vi "mbtester_main.vi"() -> ()   [LabVIEW 2012]
uses:
  source/TSKMGR_TaskManager/mbTest_main_gui_states.ctl
  <vilib>/Utility/miscctls.llb/LVRectTypeDef.ctl
  <vilib>/Utility/miscctls.llb/LVRowAndColumnTypeDef.ctl
  <vilib>/Utility/miscctls.llb/LVRowAndColumnUnsignedTypeDef.ctl
  source/APP_AppControl/APP_AppControl.lvlib
  source/TSKMGR_TaskManager/TSKMGR_TaskManager.lvlib
  source/FP_FrontPanel/FP_FrontPanel.lvlib
  source/MBUS_Modbus/MBUS_Modbus.lvlib
  source/MBT_ModbusTester/MBT_ModbusTester.lvlib
panel:
  in  "Data Format":u16(ring) items=["Decimal", "Hexadecimal", "String"]
  in  "Multicolumn Listbox":i32(listbox)
  in  "btnClear":bool
  in  "btnSaveToFile":bool
  in  "btnDisconnect":bool
  out "isConnected":bool
  in  "btnConnect":bool
  in  "Number of Regs.":u16 max=125
  in  "Starting Reg.":u16
  in  "Port":u16
  in  "IP Address":string
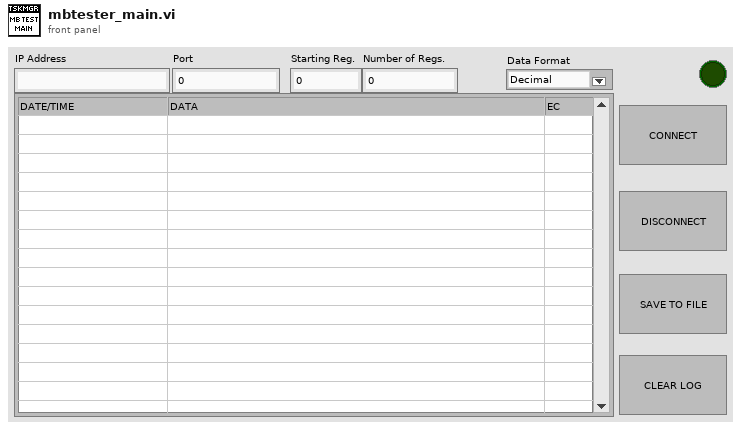
[diagram p1: front panel]
types:
  T1 = typedef "TSKMGR_TaskManager.lvlib/mbTest_main_gui_states.ctl" = enum16{"INIT", "IDLE", "CONNECT", "OPERATE", "DISCONNECT", "CLEAR", "EXIT_APP", "SAVE"}
  T2 = enum8{"Enabled", "Disabled", "Disabled and Grayed Out"}
  T3 = cluster{"isConnected":bool, "connection ID":refnum<k5>, "IP Address":string, "Port":dbl}
  T4 = typedef "LVRectTypeDef.ctl" = cluster{"Left":i16, "Top":i16, "Right":i16, "Bottom":i16}
  T5 = typedef "LVRowAndColumnUnsignedTypeDef.ctl" = cluster{"Row":u32, "Column":u32}
  T6 = typedef "LVRowAndColumnTypeDef.ctl" = cluster{"Row":i32, "Column":i32}
  T7 = cluster{"App_EvtCmds":enum16{"CLOSE_APP"}, "variant":variant}
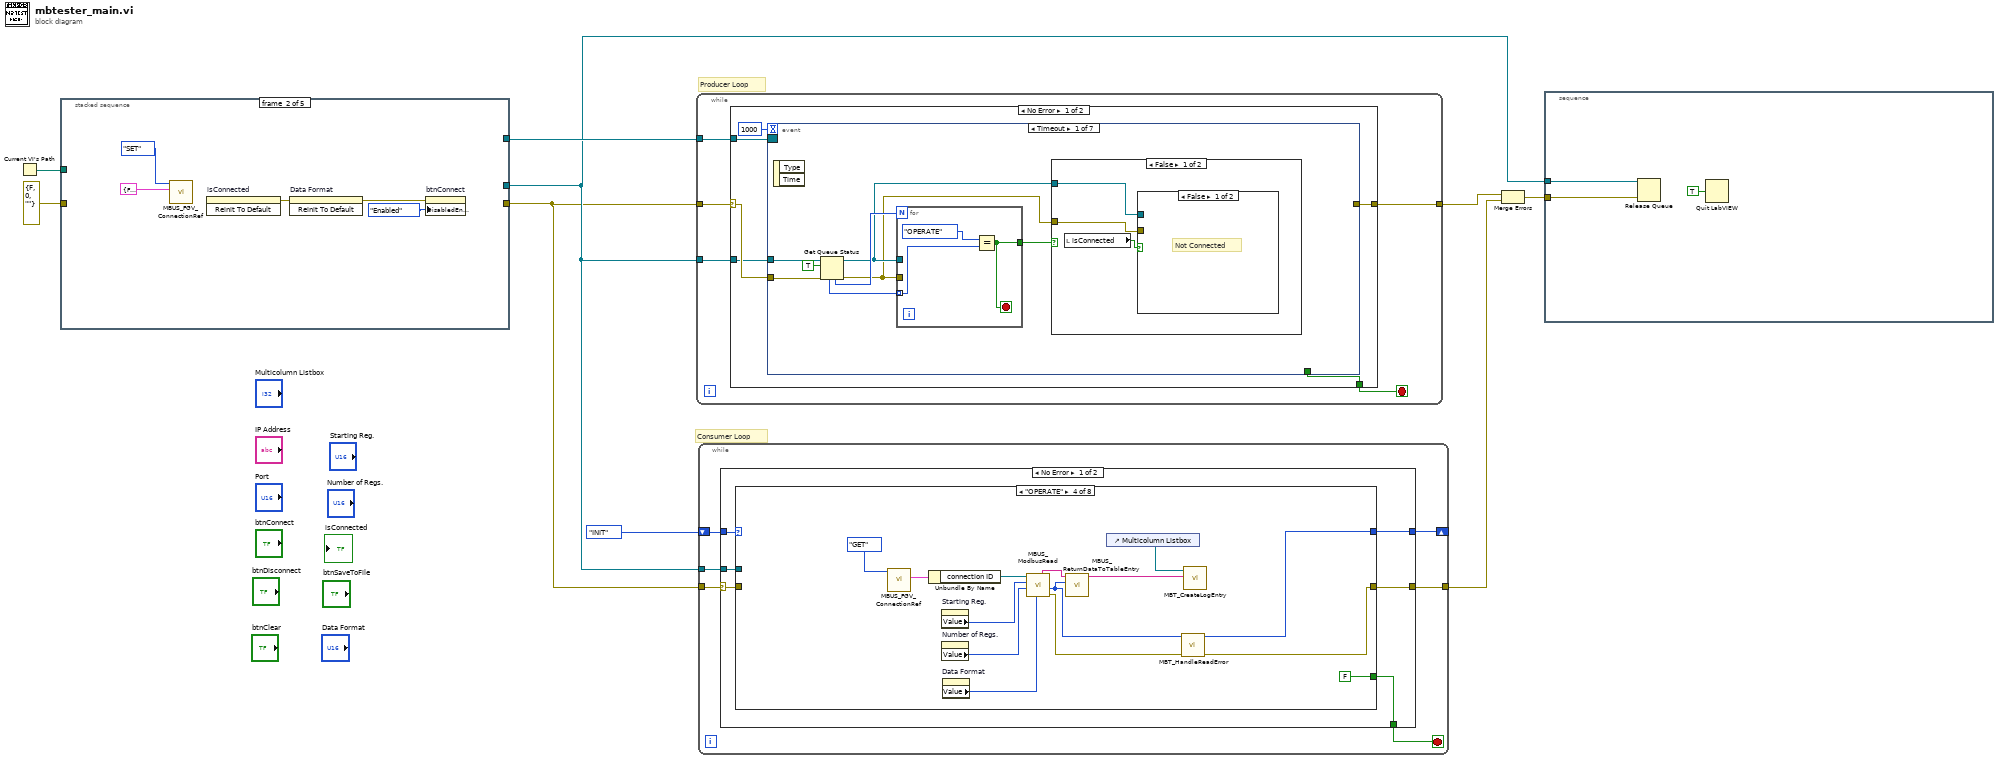
[diagram p0: block diagram]
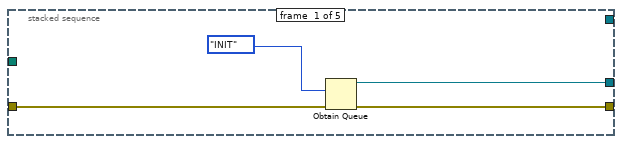
[diagram p2: hidden frame]
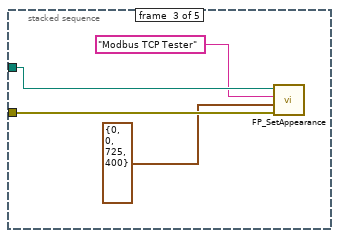
[diagram p3: hidden frame]
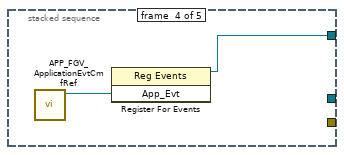
[diagram p4: hidden frame]
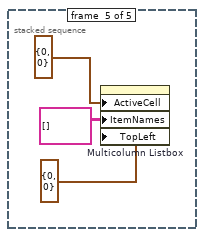
[diagram p5: hidden frame]
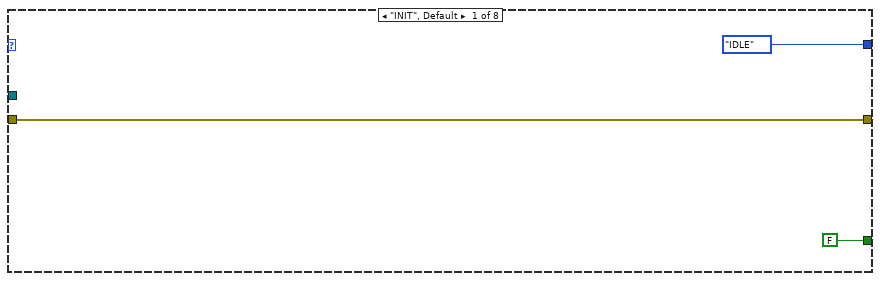
[diagram p6: hidden frame]
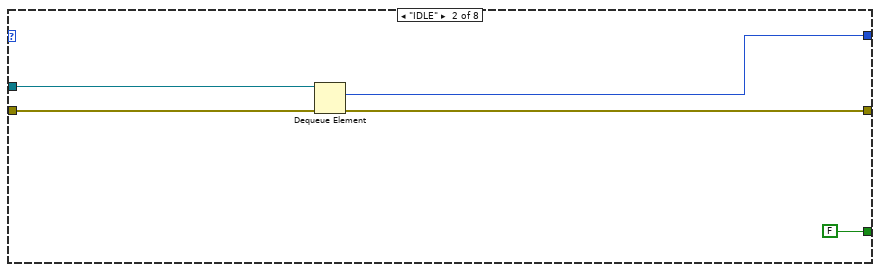
[diagram p7: hidden frame]
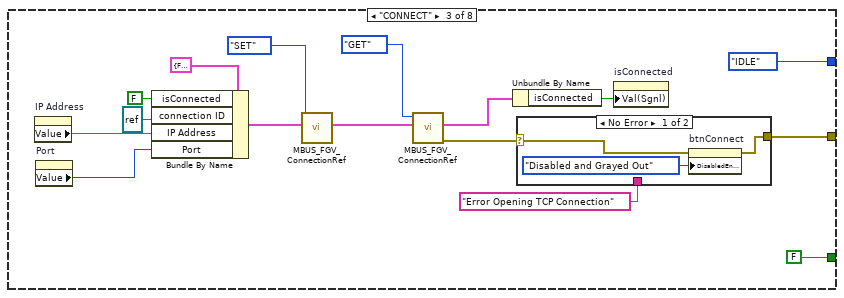
[diagram p8: hidden frame]
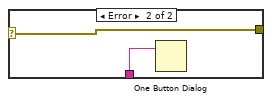
[diagram p9: hidden frame]
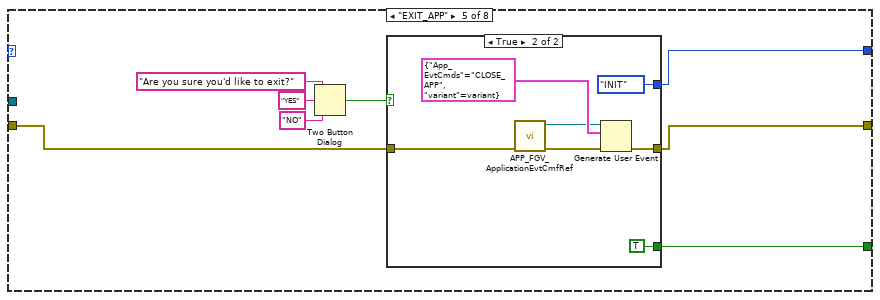
[diagram p10: hidden frame]
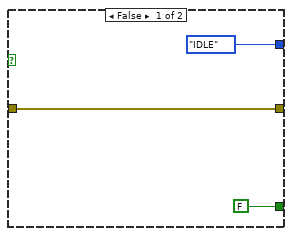
[diagram p11: hidden frame]
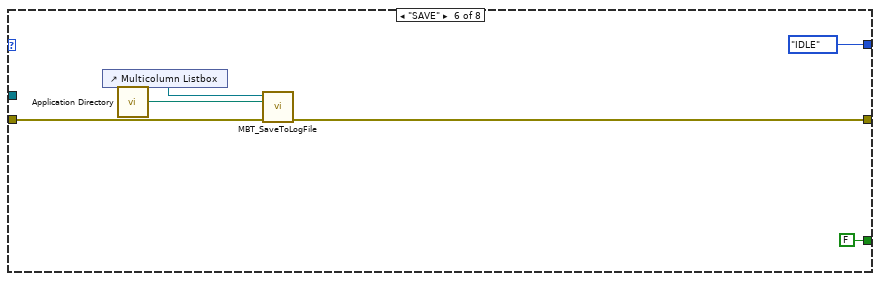
[diagram p12: hidden frame]
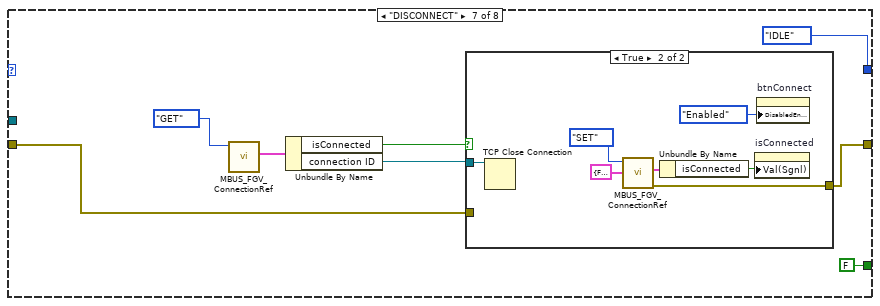
[diagram p13: hidden frame]
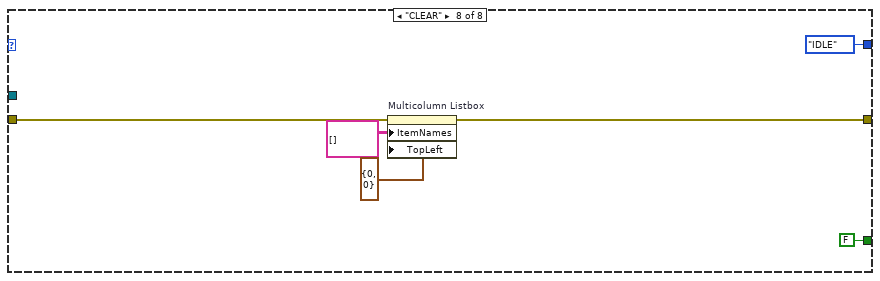
[diagram p15: hidden frame]
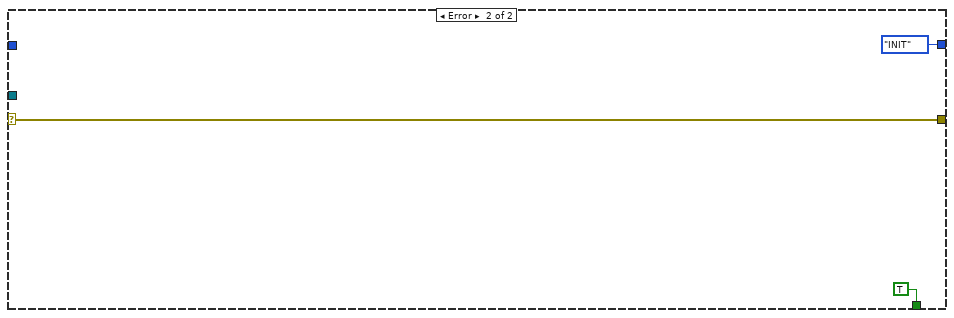
[diagram p16: hidden frame]
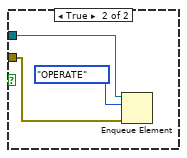
[diagram p17: hidden frame]
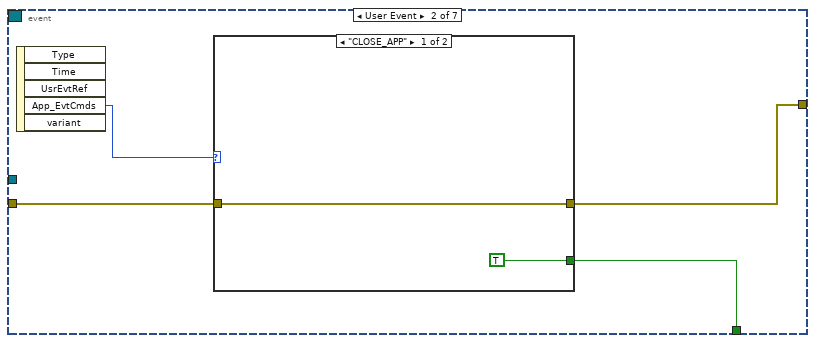
[diagram p19: hidden frame]
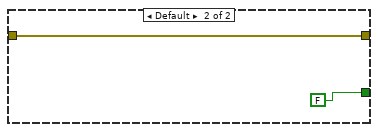
[diagram p20: hidden frame]
diagram:
  # "Consumer Loop"
  # "Producer Loop"
  n1 = Current VI's Path() -> (path=w2:path)
  n2 = stacked-sequence {
    tunnel: [_ _ _ w23 _] -> w9
    tunnel: [w10 _ _ _ _] -> w1
    tunnel: [w11 _ _ _ _] -> w3
    tunnel: errorcluster {"status"=FALSE, "code"=0, "source"=""} ("error in (no error)") -> [w13 _ w22 _ _]
    tunnel: w2 -> [_ _ w21 _ _]
    frame #0 {
      n3 = Obtain Queue(element data type=mbTest_main_gui_states."INIT", error in (no error)=w13) -> (queue out=w11:refnum<queue>, error out=w10:errorcluster)  [unwired: 3 in, 1 out]
    }
    frame #1 {
      n4 = call "MBUS_FGV_ConnectionRef.vi"("ConnectionRefIn"=T3 {"isConnected"=FALSE, "connection ID"=refnum, "IP Address"="", "Port"=0.0}, "CMD"=enum16{"GET", "SET"}."SET") -> ()  [unwired: 8 in, 2 out]
      n5 = invoke on="isConnected" class="Bool" method="Reinit To Default"() -> (error out=w14:errorcluster)  [unwired: 3 in, 2 out]
      n6 = invoke on="Data Format" class="Ring (strict)" method="Reinit To Default"(error in=w14) -> (error out=w15:errorcluster)  [unwired: 2 in, 2 out]
      n7 = property on="btnConnect" class="Bool"(error in=w15, "DisabledEnum"=T2."Enabled" ("Disabled")) -> ()  [unwired: 1 in, 2 out]
    }
    frame #2 {
      n8 = call "FP_SetAppearance.vi"("error in (no error)"=w22, "Front Panel Window:Window Bounds 2"=T4 {"Left"=0, "Top"=0, "Right"=725, "Bottom"=400}, "Front Panel Window:Title"="Modbus TCP Tester", "vi path"=w21) -> ()  [unwired: 7 in, 1 out]
    }
    frame #3 {
      n9 = call "APP_FGV_ApplicationEvtCmfRef.vi"() -> ("App_Evt"=w24:refnum<user-event>)  [unwired: 10 in, 1 out]
      n10 = register-events(w24) -> (reference out=w23:refnum<event-registration>)  [unwired: 2 in, 1 out]
    }
    frame #4 {
      n11 = property on="Multicolumn Listbox" class="MCListbox (strict)"("ActiveCell"=T6 {"Row"=0, "Column"=0} ("Active Cell:Active Cell"), "ItemNames"=string[][] [] ("Item Names"), "TopLeft"=T5 {"Row"=0, "Column"=0} ("Top Left Visible Cell")) -> ()  [unwired: 2 in, 2 out]
    }
  }
  n12 = while {
    tunnel: w9 -> [w32]
    tunnel: w1 -> [w31]
    tunnel: [w29] -> w4
    tunnel: w3 -> [w28]
    stop <- w30 stop-if-true
    n13 = case shown="No Error" w31 {
      selector: w31 -> [w37 w86]
      tunnel: w32 -> [w38 _]
      tunnel: [w34 TRUE] -> w30
      tunnel: [w36 w86] -> w29
      tunnel: w28 -> [w35 _]
      frame No Error {
        n14 = event shown="[0] Timeout" {
          selector: w38 -> [_ _ _ _ _ _ _]
          dyn-events: _ -> [_ _ _ _ _ _ _]
          timeout: 1000 -> [_ _ _ _ _ _ _]
          tunnel: w37 -> [w45 w57 w65 w70 w77 w79 w83]
          tunnel: [_ w56 _ _ w74 _ _] -> w36
          tunnel: w35 -> [w46 _ w66 w72 w76 w80 w84]
          tunnel: [_ w58 _ FALSE _ _ _] -> w34
          event Timeout {
            n15 = event-data() -> ()  [unwired: 1 in, 2 out]
            n16 = Get Queue Status(queue=w46, return elements? (F)=TRUE, error in (no error)=w45) -> (queue out=w40:refnum<queue>, error out=w39:errorcluster, # elements in queue=w44:i32, elements=w43:T1[])  [unwired: 4 out]
            n17 = for {
              N: w44 -> [_]
              tunnel: w43 -> [w49] mode=indexing
              tunnel: [w47] -> w41
              tunnel: w40 -> [_]
              tunnel: w39 -> [_]
              stop <- w47 stop-if-true
              n18 = Equal?(x=mbTest_main_gui_states."OPERATE", y=w49) -> (x = y?=w47:bool)
            }
            n19 = case shown="False" w41 {
              tunnel: w40 -> [w51 _]
              tunnel: w39 -> [w50 _]
              frame False {
                n20 = local read "isConnected"() -> (w52:bool)
                n21 = case shown="False" w52 {
                  tunnel: w51 -> [_ w54]
                  tunnel: w50 -> [_ w53]
                  frame False {
                    # "Not Connected"
                  }
                  frame True {
                    n22 = Enqueue Element(queue=w54, element=mbTest_main_gui_states."OPERATE", error in (no error)=w53) -> ()  [unwired: 1 in, 3 out]
                  }
                }
              }
              frame True {
                # "Operate already in queue"
              }
            }
          }
          event User Event {
            n23 = event-data() -> ("App_EvtCmds"=w59:enum16{"CLOSE_APP"})  [unwired: 1 in, 4 out]
            n24 = case shown="\"CLOSE_APP\"" w59 {
              tunnel: [TRUE FALSE] -> w58
              tunnel: [w60 w62] -> w56
              tunnel: w57 -> [w60 w62]
              frame "CLOSE_APP" {
              }
              frame Default {
              }
            }
          }
          event "btnClear": Value Change {
            n25 = event-data() -> ("CtlRef"=w67:refnum<vi>)  [unwired: 1 in, 4 out]
            n26 = Enqueue Element(queue=w66, element=mbTest_main_gui_states."CLEAR", error in (no error)=w65) -> ()  [unwired: 1 in, 3 out]
            n27 = invoke class="Bool" method="Reinit To Default"(reference=w67) -> ()  [unwired: 2 in, 3 out]
          }
          event "btnConnect": Value Change {
            n28 = event-data() -> ("CtlRef"=w69:refnum<vi>)  [unwired: 1 in, 4 out]
            n29 = Enqueue Element(queue=w72, element=mbTest_main_gui_states."CONNECT", error in (no error)=w70) -> ()  [unwired: 1 in, 3 out]
            n30 = invoke class="Bool" method="Reinit To Default"(reference=w69) -> ()  [unwired: 2 in, 3 out]
          }
          event Panel Close? {
            n31 = event-data() -> ()  [unwired: 1 in, 3 out]
            n32 = Enqueue Element At Opposite End(queue=w76, element=mbTest_main_gui_states."EXIT_APP", error in (no error)=w77) -> (error out=w74:errorcluster)  [unwired: 1 in, 2 out]
            n33 = event-data("Discard?"=TRUE) -> ()  [unwired: 1 in, 1 out]
          }
          event "btnDisconnect": Value Change {
            n34 = event-data() -> ("CtlRef"=w78:refnum<vi>)  [unwired: 1 in, 4 out]
            n35 = Enqueue Element(queue=w80, element=mbTest_main_gui_states."DISCONNECT", error in (no error)=w79) -> ()  [unwired: 1 in, 3 out]
            n36 = invoke class="Bool" method="Reinit To Default"(reference=w78) -> ()  [unwired: 2 in, 3 out]
          }
          event "btnSaveToFile": Value Change {
            n37 = event-data() -> ("CtlRef"=w85:refnum<vi>)  [unwired: 1 in, 4 out]
            n38 = Enqueue Element(queue=w84, element=mbTest_main_gui_states."SAVE", error in (no error)=w83) -> ()  [unwired: 1 in, 3 out]
            n39 = invoke class="Bool" method="Reinit To Default"(reference=w85) -> ()  [unwired: 2 in, 3 out]
          }
        }
      }
      frame Error {
      }
    }
  }
  n40 = while {
    tunnel: w1 -> [w93]
    tunnel: w3 -> [w91]
    shift-right: [w89] -> _
    shift-left: mbTest_main_gui_states."INIT" -> [w90]
    tunnel: [w88] -> w5
    stop <- w92 stop-if-true
    n41 = case shown="No Error" w93 {
      selector: w93 -> [w97 w190]
      tunnel: [w95 TRUE] -> w92
      tunnel: w91 -> [w94 _]
      tunnel: w90 -> [w99 _]
      tunnel: [w98 mbTest_main_gui_states."INIT"] -> w89
      tunnel: [w96 w190] -> w88
      frame No Error {
        n42 = case shown="\"OPERATE\"" w99 {
          tunnel: [mbTest_main_gui_states."IDLE" w104 mbTest_main_gui_states."IDLE" ("f") w129 w144 mbTest_main_gui_states."IDLE" mbTest_main_gui_states."IDLE" mbTest_main_gui_states."IDLE"] -> w98
          tunnel: w97 -> [w101 w106 _ _ w146 w164 w167 w186]
          tunnel: [w101 w103 w110 w130 w145 w163 w169 w185] -> w96
          tunnel: [FALSE FALSE FALSE FALSE w143 FALSE FALSE FALSE] -> w95
          tunnel: w94 -> [_ w105 _ _ _ _ _ _]
          frame "INIT", Default {
          }
          frame "IDLE" {
            n43 = Dequeue Element(queue=w105, error in (no error)=w106) -> (element=w104:T1, error out=w103:errorcluster)  [unwired: 1 in, 2 out]
          }
          frame "CONNECT" {
            n44 = property on="IP Address" class="Str"() -> ("Value"=w116:string)  [unwired: 2 in, 2 out]
            n45 = property on="Port" class="DigNum (strict)"() -> ("Value"=w115:u16)  [unwired: 2 in, 2 out]
            n46 = Bundle By Name(cluster=T3 {"isConnected"=FALSE, "connection ID"=refnum, "IP Address"="", "Port"=0.0} ("ConnectionRefIn"), "isConnected"=FALSE, "connection ID"=refnum<k5> refnum, "IP Address"=w116, "Port"=w115) -> (w119:T3)
            n47 = call "MBUS_FGV_ConnectionRef.vi"("ConnectionRefIn"=w119, "CMD"=enum16{"GET", "SET"}."SET") -> ("ConnectionRefOut"=w118:T3)  [unwired: 8 in, 1 out]
            n48 = call "MBUS_FGV_ConnectionRef.vi"("ConnectionRefIn"=w118, "CMD"=enum16{"GET", "SET"}."GET") -> ("error out"=w111:errorcluster, "ConnectionRefOut"=w117:T3)  [unwired: 8 in]
            n49 = Unbundle By Name(w117) -> ("isConnected"=w108:bool)
            n50 = case shown="No Error" w111 {
              selector: w111 -> [w125 w127]
              tunnel: [w126 w127] -> w110
              tunnel: "Error Opening TCP Connection" -> [_ w128]
              frame No Error {
                n51 = property on="btnConnect" class="Bool"(error in=w125, "DisabledEnum"=T2."Disabled and Grayed Out" ("Disabled")) -> (error out=w126:errorcluster)  [unwired: 1 in, 1 out]
              }
              frame Error {
                n52 = One Button Dialog(message=w128) -> ()  [unwired: 1 in, 1 out]
              }
            }
            n53 = property on="isConnected" class="Bool"("Val(Sgnl)"=w108) -> ()  [unwired: 2 in, 2 out]
          }
          frame "OPERATE" {
            n54 = call "MBUS_FGV_ConnectionRef.vi"("CMD"=enum16{"GET", "SET"}."GET") -> ("ConnectionRefOut"=w140:T3)  [unwired: 9 in, 1 out]
            n55 = Unbundle By Name(w140) -> ("connection ID"=w139:refnum<k5>)
            n56 = property on="Starting Reg." class="DigNum (strict)"() -> ("Value"=w138:u16)  [unwired: 2 in, 2 out]
            n57 = property on="Number of Regs." class="DigNum (strict)"() -> ("Value"=w137:u16)  [unwired: 2 in, 2 out]
            n58 = property on="Data Format" class="Ring (strict)"() -> ("Value"=w133:u16)  [unwired: 2 in, 2 out]
            n59 = call "MBUS_ModbusRead.vi"("Format"=w133, "NumRegs"=w137, "StartingAddr"=w138, "connection ID"=w139) -> ("error out"=w131:errorcluster, "ModbusExceptionCode"=w132:u8, "String_out"=w136:string)  [unwired: 3 in, 2 out]
            n60 = call "MBUS_ReturnDataToTableEntry.vi"("Exception Code"=w132, "dataIn"=w136) -> ("dataOut"=w135:string[])  [unwired: 9 in]
            n61 = control-ref of="Multicolumn Listbox"() -> (w134:refnum<vi>)
            n62 = call "MBT_HandleReadError.vi"("error in"=w131, "ModbusExceptionCode"=w132) -> ("error out"=w130:errorcluster, "state"=w129:T1)  [unwired: 8 in]
            n63 = call "MBT_CreateLogEntry.vi"("Array"=w135, "MulticolumnListbox in"=w134) -> ()  [unwired: 10 in]
          }
          frame "EXIT_APP" {
            n64 = Two Button Dialog(message="Are you sure you'd like to exit?", 1:"NO" ("F button name (\"Cancel\")"), 2:"YES" ("T button name (\"OK\")")) -> (T button?=w150:bool)
            n65 = case shown="True" w150 {
              tunnel: w146 -> [w153 w157]
              tunnel: [w153 w155] -> w145
              tunnel: [mbTest_main_gui_states."IDLE" mbTest_main_gui_states."INIT"] -> w144
              tunnel: [FALSE TRUE] -> w143
              frame False {
              }
              frame True {
                n66 = call "APP_FGV_ApplicationEvtCmfRef.vi"("error in"=w157) -> ("error out"=w158:errorcluster, "App_Evt"=w159:refnum<user-event>)  [unwired: 9 in]
                n67 = Generate User Event(user event=w159, event data cluster=T7 {"App_EvtCmds"=enum."CLOSE_APP", "variant"=variant} ("event data"), error in=w158) -> (error out=w155:errorcluster)  [unwired: 1 out]
              }
            }
          }
          frame "SAVE" {
            n68 = control-ref of="Multicolumn Listbox"() -> (w162:refnum<vi>)
            n69 = call <vilib>:"Application Directory.vi"() -> ("Application Directory"=w161:path)
            n70 = call "MBT_SaveToLogFile.vi"("error in"=w164, "path"=w161, "MulticolumnListbox in"=w162) -> ("error out"=w163:errorcluster)  [unwired: 8 in]
          }
          frame "DISCONNECT" {
            n71 = call "MBUS_FGV_ConnectionRef.vi"("CMD"=enum16{"GET", "SET"}."GET") -> ("ConnectionRefOut"=w173:T3)  [unwired: 9 in, 1 out]
            n72 = Unbundle By Name(w173) -> ("isConnected"=w172:bool, "connection ID"=w171:refnum<k5>)
            n73 = case shown="True" w172 {
              tunnel: w171 -> [_ w182]
              tunnel: [w175 w177] -> w169
              tunnel: w167 -> [w175 _]
              frame False {
              }
              frame True {
                n74 = TCP Close Connection(connection ID=w182) -> ()  [unwired: 2 in, 2 out]
                n75 = call "MBUS_FGV_ConnectionRef.vi"("ConnectionRefIn"=T3 {"isConnected"=FALSE, "connection ID"=refnum, "IP Address"="", "Port"=0.0}, "CMD"=enum16{"GET", "SET"}."SET") -> ("error out"=w177:errorcluster, "ConnectionRefOut"=w179:T3)  [unwired: 8 in]
                n76 = Unbundle By Name(w179) -> ("isConnected"=w178:bool)
                n77 = property on="isConnected" class="Bool"("Val(Sgnl)"=w178) -> ()  [unwired: 2 in, 2 out]
                n78 = property on="btnConnect" class="Bool"("DisabledEnum"=T2."Enabled" ("Disabled")) -> ()  [unwired: 2 in, 2 out]
              }
            }
          }
          frame "CLEAR" {
            n79 = property on="Multicolumn Listbox" class="MCListbox (strict)"(error in=w186, "ItemNames"=string[][] [] ("Item Names"), "TopLeft"=T5 {"Row"=0, "Column"=0} ("Top Left Visible Cell")) -> (error out=w185:errorcluster)  [unwired: 1 in, 1 out]
          }
        }
      }
      frame Error {
      }
    }
  }
  n80 = Merge Errors(w4, w5) -> (w7:errorcluster)
  n81 = stacked-sequence {
    tunnel: w3 -> [w194]
    tunnel: w7 -> [w193]
    frame #0 {
      n82 = Release Queue(queue=w194, error in (no error)=w193) -> ()  [unwired: 1 in, 3 out]
      n83 = Quit LabVIEW(quit? (T)=TRUE) -> ()
    }
  }
